vi "PH_PP_Common.set PSU Type.vi"(1 "PU":T1) -> (0 "PSU Type":T2)   [LabVIEW 2014, in "PH_PP_Common.lvlib"]
uses:
  PH_PP_Common.lvlib
  PH_PP_Common.PSU Type.ctl
  PH_PP_Common.PUs.ctl
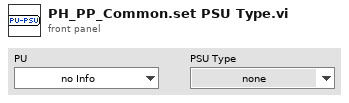
[diagram p1: front panel]
types:
  T1 = typedef "PH_PP_Common.lvlib/PH_PP_Common.PUs.ctl" = enum16{"no Info", "PA-19mm-1", "PA-19mm-2", "PA-45mm-PILC", "PA-45mm-MAIN", "MA-PU-1", "MA-PU-2", "MA-PU-3", "MA-PU-4", "MA-PU-5", "MA-PU-6", "MA-FR", "MA-PILC", "PA-45mm-DP"}
  T2 = typedef "PH_PP_Common.lvlib/PH_PP_Common.PSU Type.ctl" = enum16{"none", "Maxwell Standard", "DEL", "Maxwell ALE", "Continuum 601k"}
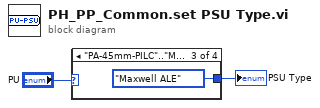
[diagram p0: block diagram]
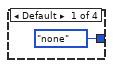
[diagram p2: hidden frame]
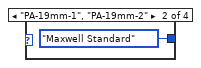
[diagram p3: hidden frame]
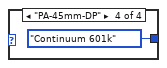
[diagram p4: hidden frame]
diagram:
  n1 = case shown="\"PA-45mm-PILC\"..\"MA-PILC\"" "PU" {
    tunnel: [PH_PP_Common.PSU_Type."none" ("PSU Type 2") PH_PP_Common.PSU_Type."Maxwell Standard" ("PSU Type 2") PH_PP_Common.PSU_Type."Maxwell ALE" ("PSU Type 2") PH_PP_Common.PSU_Type."Continuum 601k" ("PSU Type 2")] -> w2
    frame Default {
    }
    frame "PA-19mm-1", "PA-19mm-2" {
    }
    frame "PA-45mm-PILC".."MA-PILC" {
    }
    frame "PA-45mm-DP" {
    }
  }
  "PSU Type" <- w2
